vi "String_Temperature.vi"(11 "String":string="Set Temperatura 4.2K at 20K/min, FastSettle, Wait") -> (1 "T.Approach":i32(ring) items=["FastSettle", "NoOvershoot"], 2 "Rate":dbl, 3 "Temperature":dbl, 4 "T.Wait Stability":bool)   [LabVIEW 2017]
panel:
  out "subString":string
  # "Set Temperatura 4.2K at 20K/min, FastSettle, Wait"
  # "Set Temperatura 4.2K at 20K/min, FastSettle, NOWait"
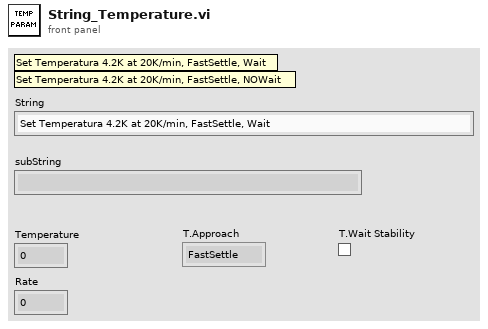
[diagram p1: front panel]
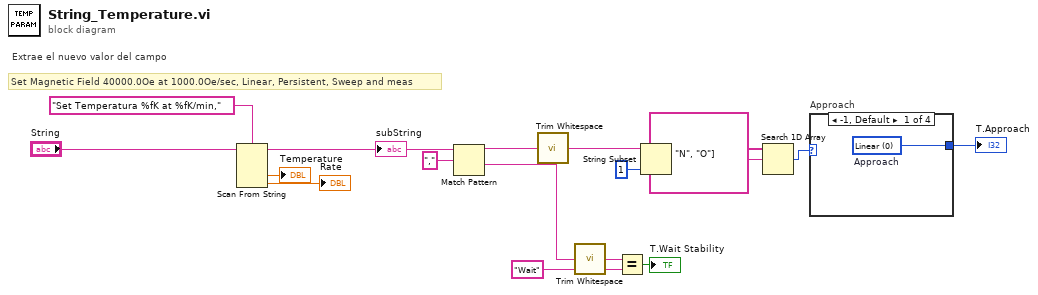
[diagram p0: block diagram]
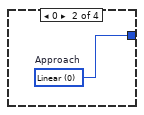
[diagram p2: hidden frame]
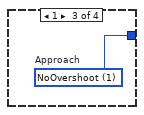
[diagram p3: hidden frame]
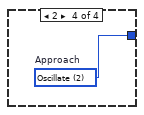
[diagram p4: hidden frame]
diagram:
  # "Set Magnetic Field 40000.0Oe at 1000.0Oe/sec, Linear, Persistent, Sweep and meas"
  # "Extrae el nuevo valor del campo"
  n1 = Scan From String(format string="Set Temperatura %fK at %fK/min,", input string="String") -> (remaining string=w2:string, output 1=→"Temperature":dbl, output 2=→"Rate":dbl)  [unwired: 4 in, 2 out]
  "subString" <- w2
  n2 = Match Pattern(string=w2, regular expression=",") -> (before substring=w5:string, after substring=w1:string)  [unwired: 1 in, 2 out]
  n3 = call <vilib>:"Trim Whitespace.vi"("string"=w5) -> ("trimmed string"=w4:string)  [unwired: 1 in]
  n4 = call <vilib>:"Trim Whitespace.vi"("string"=w1) -> ("trimmed string"=w3:string)  [unwired: 1 in]
  n5 = Equal?(x=w3, y="Wait" ("after substring")) -> (x = y?=→"T.Wait Stability":bool)
  n6 = String Subset(string=w4, length (rest)=1 ("length (rest)")) -> (substring=w12:string)  [unwired: 1 in]
  n7 = Search 1D Array(1D array=string[] ["L", "N", "O"], element=w12) -> (index of element=w11:i32)  [unwired: 1 in]
  n8 = case "Approach" shown="-1, Default" w11 {
    tunnel: [w18 w19 w20 w21] -> w10
    frame -1, Default {
      w18 = 0 items=["Linear", "NoOvershoot", "Oscillate"]  # Approach
    }
    frame 0 {
      w19 = 0 items=["Linear", "NoOvershoot", "Oscillate"]  # Approach
    }
    frame 1 {
      w20 = 1 items=["Linear", "NoOvershoot", "Oscillate"]  # Approach
    }
    frame 2 {
      w21 = 2 items=["Linear", "NoOvershoot", "Oscillate"]  # Approach
    }
  }
  "T.Approach" <- w10
